vi "SelectTubelLast.vi"(8 "error in (no error)":errorcluster, 10 "Unique Object Identifier":string, 11 "DataHandler in":refnum<class "DataHandlerMYiTOPS.lvclass">) -> (0 "error out":errorcluster, 2 "appended array":string[](array[string]), 3 "DataHandler out":refnum<class "DataHandlerMYiTOPS.lvclass">)   [LabVIEW 2017, in "DataHandlerMYiTOPS.lvclass"]
uses:
  DataHandlerMYiTOPS.lvclass
  DataHandlerMYiTOPS.lvclass/DataHandlerMYiTOPS.ctl
  <vilib>/drjdpowell/SQLite Library/SQL Statement/SQL Statement.lvclass/SQL Statement.ctl
  <vilib>/drjdpowell/SQLite Library/SQL Statement/Column I64.vi
  <vilib>/drjdpowell/SQLite Library/SQL Statement/Step.vi
  <vilib>/drjdpowell/SQLite Library/SQL Statement/Error Message.vi
  <vilib>/drjdpowell/SQLite Library/SQL Statement/Column String.vi
  <vilib>/drjdpowell/SQLite Library/SQL Statement/SQL Statement.lvclass
  <vilib>/drjdpowell/SQLite Library/SQL Connection/Connection.lvclass
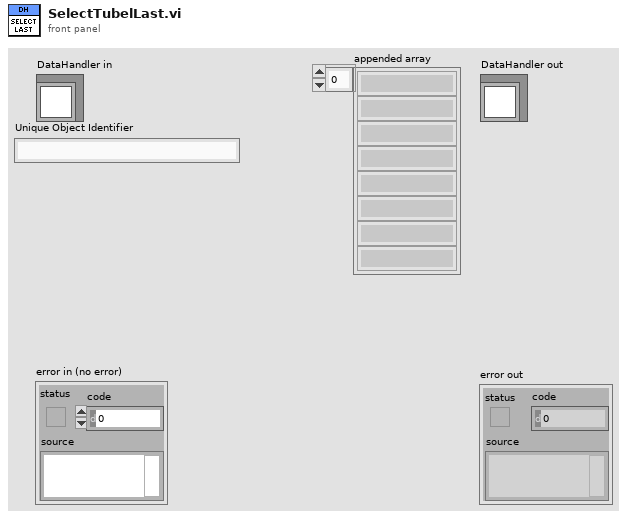
[diagram p1: front panel]
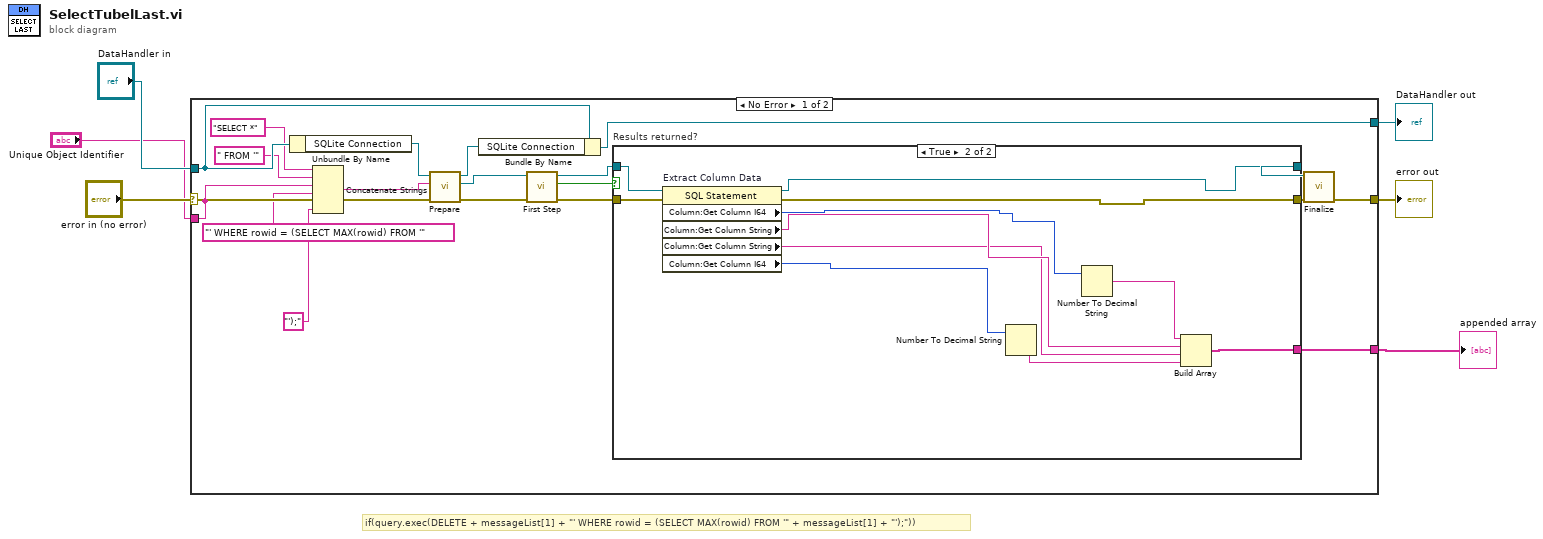
[diagram p0: block diagram]
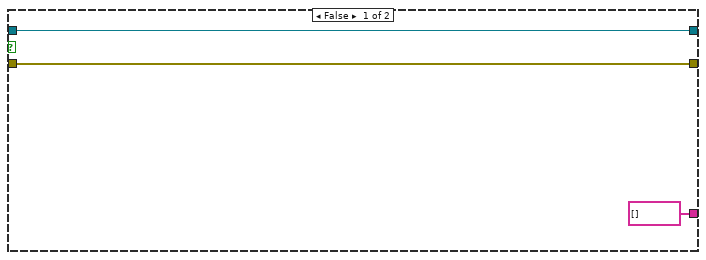
[diagram p2: hidden frame]
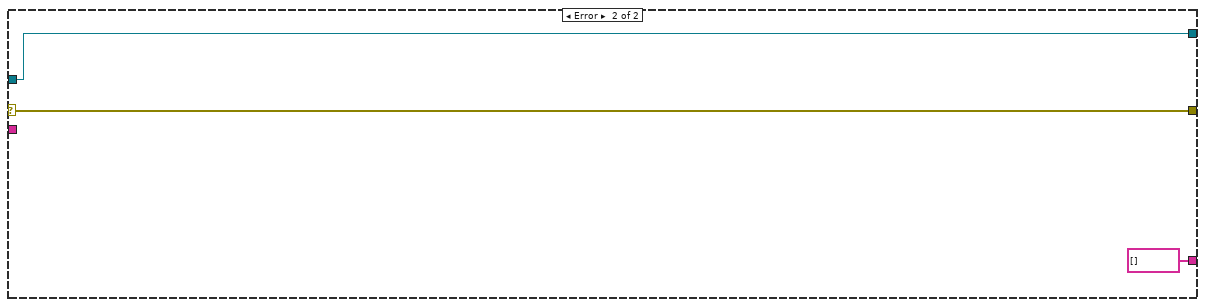
[diagram p3: hidden frame]
diagram:
  # "if(query.exec(DELETE + messageList[1] + \"' WHERE rowid = (SELECT MAX(rowid) FROM '\" + messageList[1] + \"');\"))"
  n1 = case shown="No Error" "error in (no error)" {
    selector: "error in (no error)" -> [w15 w43]
    tunnel: [w14 w43] -> w5
    tunnel: [w17 w42] -> w3
    tunnel: "DataHandler in" -> [w18 w42]
    tunnel: "Unique Object Identifier" -> [w8 _]
    tunnel: [w7 string[] []] -> w1
    frame No Error {
      n2 = Unbundle By Name(w18) -> ("SQLite Connection"=w19:refnum<class "Connection.lvclass">)
      n3 = Concatenate Strings("SELECT *" ("string"), " FROM '" ("string"), w8, "' WHERE rowid = (SELECT MAX(rowid) FROM '" ("string"), w8, "');" ("string")) -> (w12:string)
      n4 = call <vilib>:"Prepare.vi"("error in (no error)"=w15, "SQL"=w12, "SQLite Connection in"=w19) -> ("error out"=w20:errorcluster, "SQL Statement out"=w21:refnum<class "SQL Statement.lvclass">, "SQLite Connection out"=w16:refnum<class "Connection.lvclass">)  [unwired: 4 in, 2 out]
      n5 = Bundle By Name(cluster=w18, "SQLite Connection"=w16) -> (w17:refnum<class "DataHandlerMYiTOPS.lvclass">)
      n6 = call <vilib>:"First Step.vi"("error in (no error)"=w20, "SQL Statement in"=w21) -> ("error out"=w23:errorcluster, "Row returned"=w22:bool, "SQL Statement out"=w24:refnum<class "SQL Statement.lvclass">)  [unwired: 7 in]
      n7 = case "Results returned?" shown="True" w22 {
        tunnel: [w29 w32] -> w25
        tunnel: [w28 w31] -> w26
        tunnel: w24 -> [w29 w40]
        tunnel: w23 -> [w28 w39]
        tunnel: [string[] [] w30] -> w7
        frame False {
        }
        frame True {
          n8 = property on="Extract Column Data" class="SQL Statement"(reference=w40, error in=w39) -> (reference out=w32:refnum<class "SQL Statement.lvclass">, error out=w31:errorcluster, "Column:Get Column I64"=w35:i64, "Column:Get Column String"=w36:string, "Column:Get Column String"=w33:string, "Column:Get Column I64"=w38:i64)
          n9 = Number To Decimal String(number=w38) -> (decimal integer string=w37:string)  [unwired: 1 in]
          n10 = Number To Decimal String(number=w35) -> (decimal integer string=w34:string)  [unwired: 1 in]
          n11 = Build Array(w34, w36, w33, w37) -> (w30:string[])
        }
      }
      n12 = call <vilib>:"Finalize.vi"("error in (no error)"=w26, "SQL Statement in"=w25) -> ("error out"=w14:errorcluster)  [unwired: 9 in]
    }
    frame Error {
    }
  }
  "error out" <- w5
  "DataHandler out" <- w3
  "appended array" <- w1
